vi "FestoCPX.File.Read.vi"(8 "error in":errorcluster, 11 "Settings dir":path) -> (0 "error out":errorcluster)   [LabVIEW 2016]
uses:
  FestoCPX.DO.Signal.ctl
  FestoCPX.DI.Signal.ctl
  FestoCPX.DI.ctl
  FestoCPX.DO.ctl
  FestoCPX.DI.Sets.ctl
  FestoCPX.DO.Sets.ctl
  FestoCPX.Global.vi
  <vilib>/Utility/config.llb/Read Key (String).vi
  <vilib>/Utility/config.llb/Read Key (I32).vi
  Global/ApplicationGlobal.vi
  <vilib>/Utility/config.llb/NI_LVConfig.lvlib
panel:
  in  "DO":T1
  in  "DI":T2=enum."1.0"
  in  "DI Signal":T3
  in  "DO Signal":T4
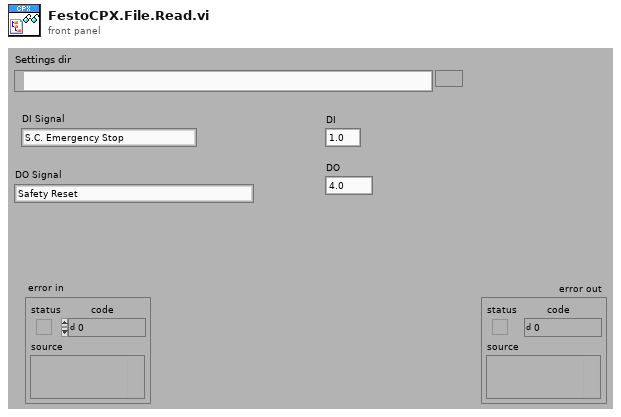
[diagram p1: front panel]
types:
  T1 = typedef "FestoCPX.DO.ctl" = enum16{"4.0", "4.1", "4.2", "4.3", "4.4", "4.5", "4.6", "4.7", "5.0", "5.1", "5.2", "5.3", "5.4", "5.5", "5.6", "5.7", "6.0", "6.1", "6.2", "6.3", "6.4", "6.5", "6.6", "6.7", "Q1K1", "Q1K2", "Q2K1", "Q2K2", "Q3K1", "Q3K2", "Q4K1", "Q4K2", "Q5K1", "Q5K2", "Q6K1", "Q6K2"}
  T2 = typedef "FestoCPX.DI.ctl" = enum16{"0.0", "0.1", "0.2", "0.3", "0.4", "0.5", "0.6", "0.7", "1.0", "1.1", "1.2", "1.3", "1.4", "1.5", "1.6", "1.7", "2.0", "2.1", "2.2", "2.3", "2.4", "2.5", "2.6", "2.7", "3.0", "3.1", "3.2", "3.3", "3.4", "3.5", "3.6", "3.7", "4.0", "4.1", "4.2", "4.3", "4.4", "4.5", "4.6", "4.7"}
  T3 = typedef "FestoCPX.DI.Signal.ctl" = enum16{"S.C. Emergency Stop", "S.C. Side Door Close", "S.C. Front Door Close", "S.C. Front Door Secured", "Button Start", "Button Stop", "Button Control", "Product Move Home", "Product Move Work", "Table Position", "Table Lock", "Product Lift A Home", "Product Lift B Home", "Product Arm OK", "Product Arm NOK", "Product Arm Work", "Revolver ID 1", "Revolver ID 2", "Revolver ID 3", "Revolver ID 4", "Revolver ID 5", "Air Pressure Inside", "Air Pressure Inlet", "Product Slot 1 A Present", "Product Slot 1 B Present", "Product Slot 2 A Present", "Product Slot 2 B Present", "Product Slot 3 A Present", "Product Slot 3 B Present", "Product Slot 4 A Present", "Product Slot 4 B Present", "Product Final A Present", "Product Final B Present", "Product Output A Present", "Product Output B Present", "Product Container OK Present", "Product Container NOK Present", "Fork ID 1", "Fork ID 2"}
  T4 = typedef "FestoCPX.DO.Signal.ctl" = enum16{"Safety Reset", "Air Main Valve", "Door Lock", "Button LED Start", "Button LED Stop", "Button LED Control", "Traffic LED Red", "Traffic LED Orange", "Traffic LED Green", "Horn", "Laser Interlock", "Laser Trigger", "Laser Fume Extractor", "Product Suction Gripper Slot 1 A", "Product Suction Gripper Slot 1 B", "Product Suction Gripper Slot 2 A", "Product Suction Gripper Slot 2 B", "Product Suction Gripper Slot 3 A", "Product Suction Gripper Slot 3 B", "Product Suction Gripper Slot 4 A", "Product Suction Gripper Slot 4 B", "Product Suction Gripper Final A", "Product Suction Gripper Final B", "Lamp", "Q1 Product Move Work", "Q1 Product Move Home", "Q2 Table Turn Work", "Q2 Table Turn Home", "Q3 Product Lift A", "Q3 Product Lift B", "Q4 Product Arm OK", "Q4 Product Arm NOK", "Q5 Product Arm Work", "Q6 Product BlowOut A", "Q6 Product BlowOut B"}
  T5 = typedef "FestoCPX.DI.Sets.ctl" = cluster{"Name":string, "Channel":T2, "Negate":bool}
  T6 = typedef "FestoCPX.DO.Sets.ctl" = cluster{"Name":string, "Channel":T1, "Negate":bool, "Default":bool}
  T7 = typedef "FestoCPX.Data.Sets.ctl" = cluster{"IP":string, "Timeout_ms":i32, "ReconnectPeriod_s":i32, "Config.DI":T5[], "Config.DO":T6[]}
  T8 = typedef "NI_LVConfig.lvlib/Config Data RefNum.ctl" = refnum<k1>
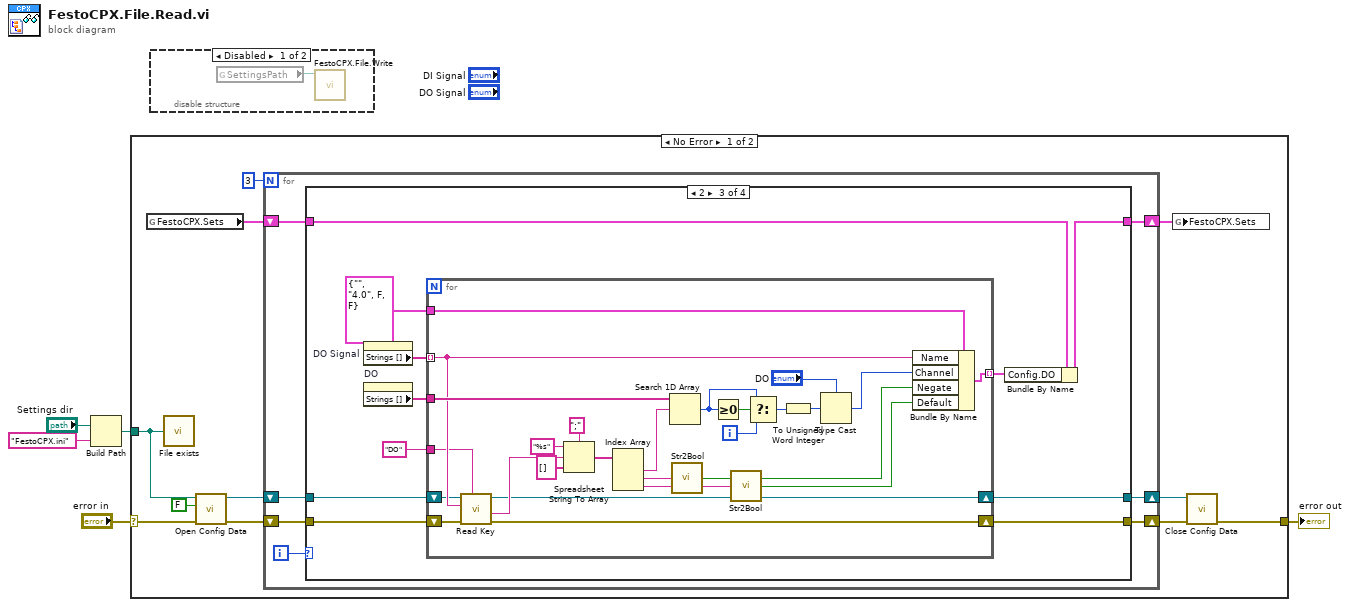
[diagram p0: block diagram]
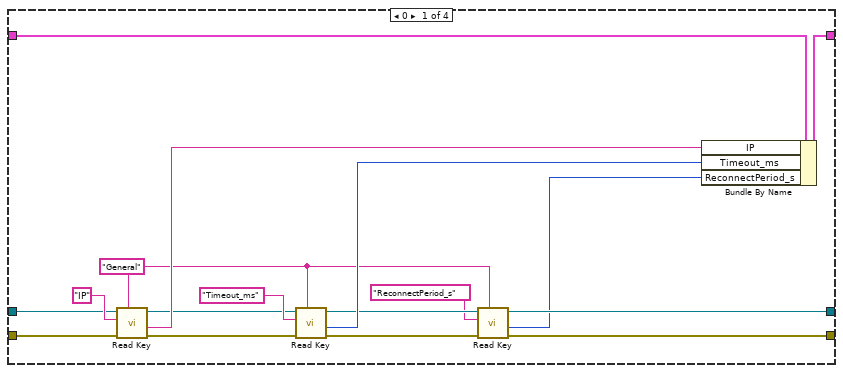
[diagram p3: hidden frame]
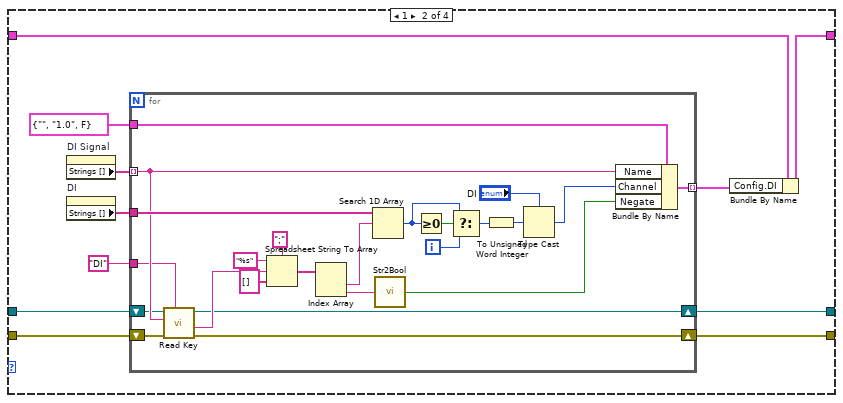
[diagram p4: hidden frame]
diagram:
  n1 = Build Path(base path="Settings dir", name or relative path="FestoCPX.ini") -> (appended path=w1:path)
  n2 = case shown="No Error" "error in" {
    selector: "error in" -> [w16 w116]
    tunnel: [w9 w116] -> w5
    tunnel: w1 -> [w15 _]
    frame No Error {
      n3 = global read "FestoCPX.Global.vi" "FestoCPX.Sets"() -> (w12:T7)
      n4 = call "File exists.vi"("file path"=w15) -> ()  [unwired: 4 in, 1 out]
      n5 = call <vilib>:"Open Config Data.vi"("error in (no error)"=w16, "create file if necessary (T)"=FALSE, "configuration file path"=w15) -> ("error out"=w14:errorcluster, "refnum"=w13:T8)  [unwired: 6 in, 1 out]
      n6 = for {
        N: 3 -> [_]
        shift-right: [w18] -> w10
        shift-left: w13 -> [w22]
        shift-right: [w21] -> w11
        shift-left: w14 -> [w23]
        shift-right: [w20] -> w8
        shift-left: w12 -> [w19]
        i -> [w17]
        n7 = case shown="2" w17 {
          tunnel: w23 -> [w40 w51 w86 w115]
          tunnel: w22 -> [w35 w49 w84 w113]
          tunnel: [w27 w46 w81 w115] -> w21
          tunnel: [w37 w43 w78 w114] -> w20
          tunnel: w19 -> [w36 w44 w79 w114]
          tunnel: [w28 w41 w76 w113] -> w18
          frame 0 {
            w26 = "General" ("section")
            n8 = call-poly <vilib>:"Read Key.vi"("section"=w26, "error in (no error)"=w40, "key"="IP", "refnum"=w35) -> ("error out"=w32:errorcluster, "value"=w39:string, "refnum out"=w33:T8)  [unwired: 4 in, 1 out]
            n9 = call-poly <vilib>:"Read Key.vi"("section"=w26, "error in (no error)"=w32, "key"="Timeout_ms", "refnum"=w33) -> ("error out"=w30:errorcluster, "value"=w31:i32, "refnum out"=w29:T8)  [unwired: 4 in, 1 out]
            n10 = call-poly <vilib>:"Read Key.vi"("section"=w26, "error in (no error)"=w30, "key"="ReconnectPeriod_s", "refnum"=w29) -> ("error out"=w27:errorcluster, "value"=w24:i32, "refnum out"=w28:T8)  [unwired: 4 in, 1 out]
            n11 = Bundle By Name(cluster=w36, "IP"=w39, "Timeout_ms"=w31, "ReconnectPeriod_s"=w24) -> (w37:T7)
          }
          frame 1 {
            n12 = property on="DI Signal" class="Enum (strict)"() -> ("Strings []"=w50:string[])  [unwired: 2 in, 2 out]
            n13 = property on="DI" class="Enum (strict)"() -> ("Strings []"=w47:string[])  [unwired: 2 in, 2 out]
            n14 = for {
              tunnel: w50 -> [w57] mode=indexing
              tunnel: T5 {"Name"="", "Channel"=enum."1.0", "Negate"=FALSE} ("DI.Sets") -> [w74]
              tunnel: w47 -> [w68]
              shift-right: [w56] -> w46
              shift-left: w51 -> [w75]
              shift-right: [w52] -> w41
              shift-left: w49 -> [w53]
              tunnel: [w55] -> w42 mode=indexing
              tunnel: "DI" ("section") -> [w54]
              i -> [w64]
              n15 = call-poly <vilib>:"Read Key.vi"("section"=w54, "error in (no error)"=w75, "key"=w57, "refnum"=w53) -> ("error out"=w56:errorcluster, "value"=w73:string, "refnum out"=w52:T8)  [unwired: 4 in, 1 out]
              n16 = Spreadsheet String To Array(delimiter (Tab)=";", format string="%s", spreadsheet string=w73, array type (2D Dbl)=string[] []) -> (array=w70:string[])
              n17 = Index Array(array=w70) -> (element #1=w67:string, element #2=w59:string)  [unwired: 2 in]
              n18 = Search 1D Array(1D array=w68, element=w67) -> (index of element=w66:i32)  [unwired: 1 in]
              n19 = call "Str2Bool.vi"("string"=w59) -> ("Boolean"=w58:bool)
              n20 = Greater Or Equal To 0?(x=w66) -> (x >= 0?=w65:bool)
              n21 = Select(t=w66, s=w65, f=w64) -> (s? t:f=w63:i32)
              n22 = To Unsigned Word Integer(number=w63) -> (unsigned 16bit integer=w62:u16)
              n23 = Type Cast(type="DI", x=w62) -> (*(type *) &x=w60:T2)
              n24 = Bundle By Name(cluster=w74, "Name"=w57, "Channel"=w60, "Negate"=w58) -> (w55:T5)
            }
            n25 = Bundle By Name(cluster=w44, "Config.DI"=w42) -> (w43:T7)
          }
          frame 2 {
            n26 = property on="DO Signal" class="Enum (strict)"() -> ("Strings []"=w85:string[])  [unwired: 2 in, 2 out]
            n27 = property on="DO" class="Enum (strict)"() -> ("Strings []"=w82:string[])  [unwired: 2 in, 2 out]
            n28 = for {
              tunnel: w85 -> [w95] mode=indexing
              tunnel: T6 {"Name"="", "Channel"=enum."4.0", "Negate"=FALSE, "Default"=FALSE} ("DO.Sets") -> [w111]
              tunnel: w82 -> [w105]
              shift-right: [w94] -> w81
              shift-left: w86 -> [w112]
              shift-right: [w89] -> w76
              shift-left: w84 -> [w90]
              tunnel: [w93] -> w77 mode=indexing
              tunnel: "DO" ("section") -> [w92]
              i -> [w101]
              n29 = call-poly <vilib>:"Read Key.vi"("section"=w92, "error in (no error)"=w112, "key"=w95, "refnum"=w90) -> ("error out"=w94:errorcluster, "value"=w110:string, "refnum out"=w89:T8)  [unwired: 4 in, 1 out]
              n30 = Spreadsheet String To Array(delimiter (Tab)=";", format string="%s", spreadsheet string=w110, array type (2D Dbl)=string[] []) -> (array=w107:string[])
              n31 = Index Array(array=w107) -> (element #1=w104:string, element #2=w97:string, element #3=w88:string)  [unwired: 3 in]
              n32 = Search 1D Array(1D array=w105, element=w104) -> (index of element=w103:i32)  [unwired: 1 in]
              n33 = call "Str2Bool.vi"("string"=w97) -> ("Boolean"=w96:bool)
              n34 = Greater Or Equal To 0?(x=w103) -> (x >= 0?=w102:bool)
              n35 = call "Str2Bool.vi"("string"=w88) -> ("Boolean"=w87:bool)
              n36 = Select(t=w103, s=w102, f=w101) -> (s? t:f=w100:i32)
              n37 = To Unsigned Word Integer(number=w100) -> (unsigned 16bit integer=w99:u16)
              n38 = Type Cast(type="DO", x=w99) -> (*(type *) &x=w98:T1)
              n39 = Bundle By Name(cluster=w111, "Name"=w95, "Channel"=w98, "Negate"=w96, "Default"=w87) -> (w93:T6)
            }
            n40 = Bundle By Name(cluster=w79, "Config.DO"=w77) -> (w78:T7)
          }
          frame Default {
          }
        }
      }
      n41 = global write "FestoCPX.Global.vi" "FestoCPX.Sets"(w8) -> ()
      n42 = call <vilib>:"Close Config Data.vi"("error in (no error)"=w11, "refnum"=w10) -> ("error out"=w9:errorcluster)  [unwired: 8 in, 1 out]
    }
    frame Error {
    }
  }
  "error out" <- w5
  n43 = disable-structure shown="Disabled" {
    frame Disabled {
      n44 = global read "ApplicationGlobal.vi" "SettingsPath"() -> (w117:path)
      n45 = call "FestoCPX.File.Write.vi"("Settings dir"=w117) -> ()  [unwired: 10 in, 1 out]
    }
    frame Enabled {
    }
  }
